vi "Path Package Type.vi"(11 "Path":path) -> (1 "Root Folder":path, 2 "Matched":bool, 3 "First Match":refnum<class "PackageAbstract.lvclass">, 4 "Available Types":string[](array[string]))   [LabVIEW 2020, in "GPack.lvlib"]
uses:
  GPack.lvlib
  PackageAbstract/PackageAbstract.lvclass
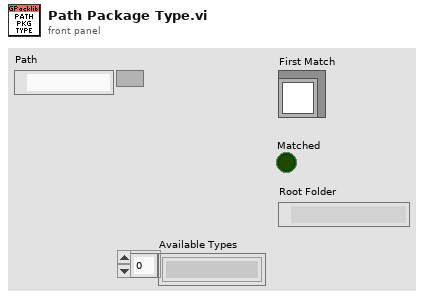
[diagram p1: front panel]
types:
  T1 = map{string, refnum<class "PackageAbstract.lvclass">}
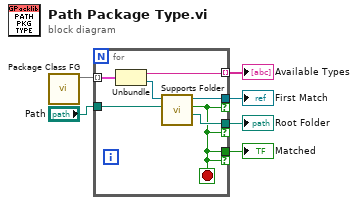
[diagram p0: block diagram]
diagram:
  n1 = call "Package Class FG.vi"() -> ("Package Classes"=w6:T1)  [unwired: 9 in, 2 out]
  n2 = for {
    tunnel: w6 -> [w13] mode=indexing
    tunnel: "Path" -> [w11]
    tunnel: [w7] -> w2 if=w7
    tunnel: [w10] -> w3 if=w7
    tunnel: [w9] -> w4 mode=indexing
    tunnel: [w8] -> w1 if=w7
    stop <- w7 stop-if-true
    n3 = Unbundle(w13) -> (w9:string, "GPack.lvlib:PackageAbstract.lvclass"=w12:refnum<class "PackageAbstract.lvclass">)
    n4 = call-dynamic "Supports Folder.vi"("Folder"=w11, "Package in"=w12) -> ("Root Folder"=w8:path, "Supported"=w7:bool, "Package out"=w10:refnum<class "PackageAbstract.lvclass">)  [unwired: 6 in, 1 out]
  }
  "Available Types" <- w4
  "First Match" <- w3
  "Matched" <- w2
  "Root Folder" <- w1
